vi "Task Read Analog.vi"(5 "Sample Rate":dbl=50.0, 7 "Samples Per Channel":i32=50, 8 "error in":errorcluster, 9 "Channel Names":string[](array[string]), 10 "Physical Channels":tag[](array[tag]), 11 "Timing Mode":i32(ring)=16097 items=["Automatic"=16097, "High Resolution"=10195, "High Speed"=14712, "Best 50 Hz Rejection"=14713, "Best 60 Hz Rejection"=14714, "Custom"=10137]) -> (0 "error out":errorcluster, 2 "data":waveform(dbl)[](array[waveform]), 3 "task out":refnum<k21>)   [LabVIEW 2020]
uses:
  <vilib>/DAQmx/read.llb/DAQmx Read (Analog 1D Wfm NChan NSamp).vi
  <vilib>/DAQmx/create/channels.llb/DAQmx Create Channel (AI-Temperature-Thermocouple).vi
  <vilib>/DAQmx/configure/timing.llb/DAQmx Timing (Sample Clock).vi
  <vilib>/DAQmx/miscellaneous.llb/DAQmx Fill In Error Info.vi
  <resource>/objmgr/daqmx.rc
panel:
  in  "Reinitialize":bool
  in  "Sample Mode":i32(ring)=10123 items=["Finite Samples"=10178, "Continuous Samples"=10123, "Hardware Timed Single Point"=12522]
  in  "Stop":bool
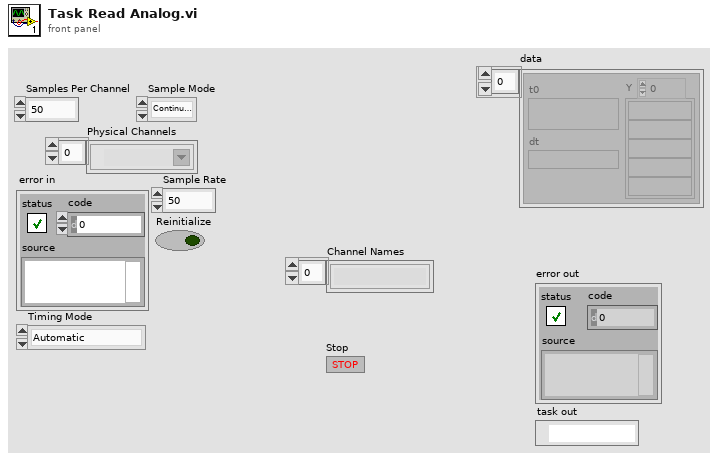
[diagram p1: front panel]
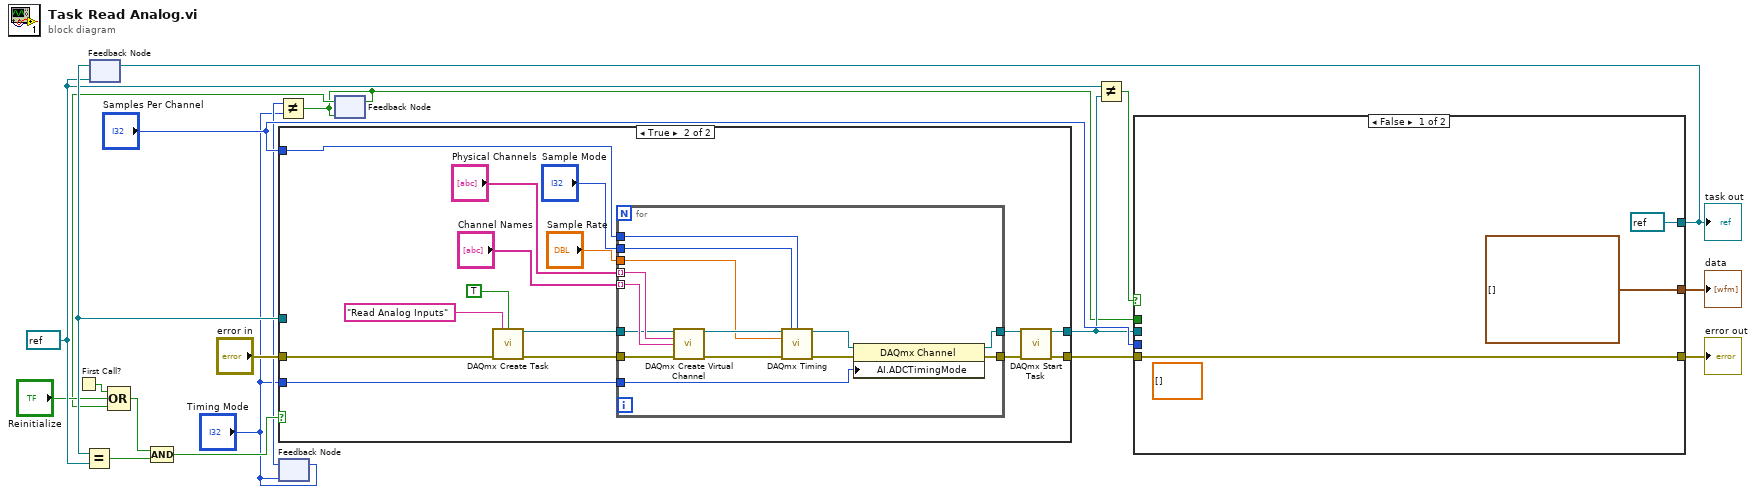
[diagram p0: block diagram]
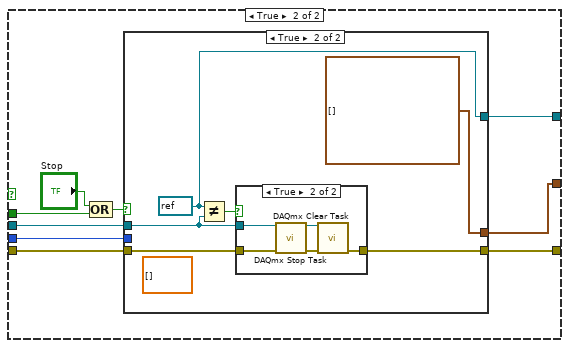
[diagram p2: hidden frame]
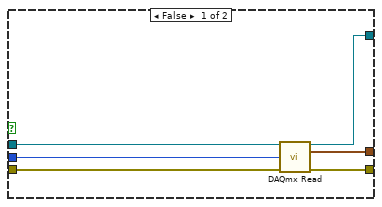
[diagram p3: hidden frame]
diagram:
  w11 = refnum<k21> refnum ("task out")
  n1 = First Call?() -> (First Call?: T/F=w6:bool)
  n2 = feedback #1(w11) -> (w12:refnum<k21>)
  n3 = Equal?(x=w12, y=w11) -> (x = y?=w10:bool)
  n4 = feedback-in #2("Timing Mode") -> ()
  n5 = feedback #2("Timing Mode") -> (w8:i32)
  n6 = Not Equal?(x=w8, y="Timing Mode") -> (x != y?=w2:bool)
  n7 = feedback-in #3(w2) -> ()
  n8 = feedback #3(w2) -> (w3:bool)
  n9 = Compound Arithmetic op=OR(w6, "Reinitialize", w3) -> (w4:bool)
  n10 = Compound Arithmetic op=AND(w4, w10) -> (w9:bool)
  n11 = case shown="True" w9 {
    tunnel: "Samples Per Channel" -> [_ w36]
    tunnel: [w20 w33] -> w13
    tunnel: [w21 w32] -> w17
    tunnel: "error in" -> [w21 w31]
    tunnel: w12 -> [w20 _]
    tunnel: "Timing Mode" -> [_ w26]
    frame False {
    }
    frame True {
      n12 = call <vilib>:"DAQmx Create Task.vi"("new task name"="Read Analog Inputs", "auto cleanup"=TRUE, "error in"=w31) -> ("task out"=w30:refnum<k21>, "error out"=w29:errorcluster)  [unwired: 11 in]
      n13 = for {
        tunnel: "Physical Channels" -> [w50] mode=indexing
        tunnel: "Channel Names" -> [w49] mode=indexing
        tunnel: w29 -> [w48]
        tunnel: "Sample Mode" -> [w45]
        tunnel: w36 -> [w44]
        tunnel: "Sample Rate" -> [w43]
        tunnel: [w38] -> w34
        tunnel: w30 -> [w47]
        tunnel: [w40] -> w35
        tunnel: w26 -> [w37]
        n14 = call-poly <vilib>:"DAQmx Create Virtual Channel.vi"("task in"=w47, "physical channels"=w50, "name to assign"=w49, "error in"=w48) -> ("task out"=w46:refnum<k21>, "error out"=w42:errorcluster)  [unwired: 10 in]
        n15 = call-poly <vilib>:"DAQmx Timing.vi"("task/channels in"=w46, "sample mode"=w45, "samples per channel"=w44, "rate"=w43, "error in"=w42) -> ("task out"=w41:refnum<k21>, "error out"=w39:errorcluster)  [unwired: 9 in]
        n16 = property class="DAQmx Channel"(reference=w41, error in=w39, "AI.ADCTimingMode"=w37) -> (reference out=w40:refnum<k21>, error out=w38:errorcluster)
      }
      n17 = call <vilib>:"DAQmx Start Task.vi"("task/channels in"=w35, "error in"=w34) -> ("task out"=w33:refnum<k21>, "error out"=w32:errorcluster)  [unwired: 12 in]
    }
  }
  n18 = Not Equal?(x=w11, y=w13) -> (x != y?=w14:bool)
  n19 = case shown="False" w14 {
    tunnel: [w52 w62] -> w19
    tunnel: "Samples Per Channel" -> [_ w61]
    tunnel: w17 -> [w52 w60]
    tunnel: w13 -> [_ w59]
    tunnel: [refnum<k21> refnum ("task out") w58] -> w15
    tunnel: w2 -> [_ w55]
    tunnel: [waveform(dbl)[] [] ("data") w54] -> w1
    frame False {
      (unwired) dbl[][] [] ("data")
    }
    frame True {
      n20 = Compound Arithmetic op=OR("Stop", w55) -> (w56:bool)
      n21 = case shown="True" w56 {
        tunnel: [w66 w71] -> w58
        tunnel: [w65 w74] -> w62
        tunnel: w59 -> [w64 w70]
        tunnel: w61 -> [w68 _]
        tunnel: w60 -> [w67 w73]
        tunnel: [w63 waveform(dbl)[] [] ("data")] -> w54
        frame False {
          n22 = call-poly <vilib>:"DAQmx Read.vi"("task/channels in"=w64, "number of samples per channel"=w68, "error in"=w67) -> ("task out"=w66:refnum<k21>, "data"=w63:waveform(dbl)[], "error out"=w65:errorcluster)  [unwired: 10 in]
        }
        frame True {
          (unwired) dbl[][] [] ("data")
          w71 = refnum<k21> refnum ("task out")
          n23 = Not Equal?(x=w71, y=w70) -> (x != y?=w72:bool)
          n24 = case shown="True" w72 {
            tunnel: [w75 w78] -> w74
            tunnel: w70 -> [_ w77]
            tunnel: w73 -> [w75 w76]
            frame False {
            }
            frame True {
              n25 = call <vilib>:"DAQmx Stop Task.vi"("task/channels in"=w77, "error in"=w76) -> ("task out"=w80:refnum<k21>, "error out"=w79:errorcluster)  [unwired: 12 in]
              n26 = call <vilib>:"DAQmx Clear Task.vi"("task in"=w80, "error in"=w79) -> ("error out"=w78:errorcluster)  [unwired: 13 in]
            }
          }
        }
      }
    }
  }
  "error out" <- w19
  "task out" <- w15
  "data" <- w1
  n27 = feedback-in #1(w15) -> ()
